vi "GetPaneRefFromLabel.vi"(8 "error in (no error)":errorcluster, 10 "Label":string, 11 "PentaPanesGUI in":refnum<class "PentaPanes.lvclass">) -> (0 "error out":errorcluster, 1 "Index (-1 not found)":i32, 2 "PaneRef":refnum<vi>, 3 "PentaPanesGUI out":refnum<class "PentaPanes.lvclass">)   [LabVIEW 2022 SP3, in "PentaPanesLibrary.lvlib" / "PentaPanes.lvclass"]
doc: "This VI reads the Pane's position string and Label.\n\nPaneRef - A reference to the pane. \nPos String - Outputs a position string (\"Top\", \"Left\", \"Right\", \"Bottom\").\nLabel.Text - Outputs The Label of the pane."
uses:
  PentaPanes.lvclass
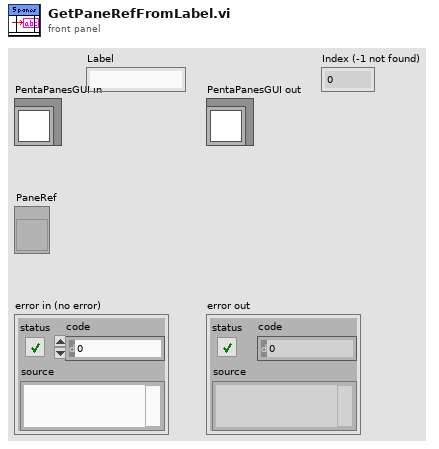
[diagram p1: front panel]
types:
  T1 = typedef "PentaPanesLibrary.lvlib/PentaPanes.lvclass/PanesCluster.ctl" = cluster{"Top Pane":refnum<vi>, "Left Pane":refnum<vi>, "Center Pane":refnum<vi>, "Right Pane":refnum<vi>, "Bottom Pane":refnum<vi>}
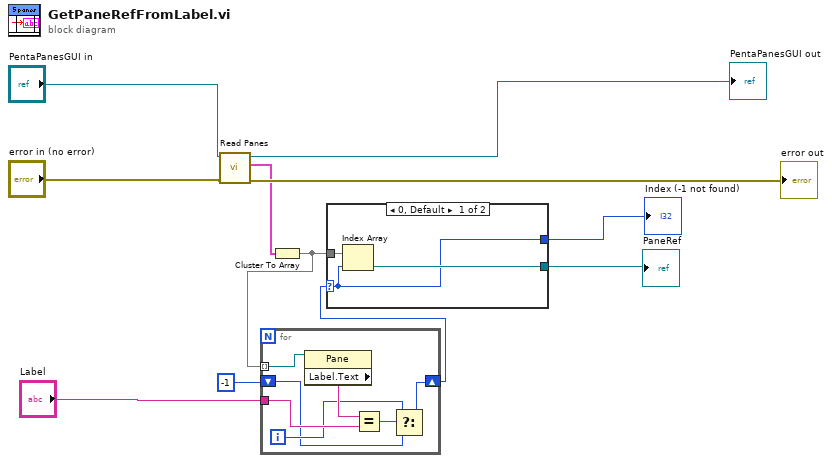
[diagram p0: block diagram]
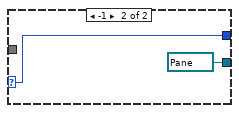
[diagram p2: hidden frame]
diagram:
  n1 = call-dynamic "Read Panes.vi"("error in (no error)"="error in (no error)", "PentaPanesGUI in"="PentaPanesGUI in") -> ("error out"=→"error out":errorcluster, "Panes"=w9:T1, "PentaPanesGUI out"=→"PentaPanesGUI out":refnum<class "PentaPanes.lvclass">)  [unwired: 7 in]
  n2 = Cluster To Array(cluster=w9) -> (array=w6:refnum<vi>[])
  n3 = for {
    tunnel: w6 -> [w18] mode=indexing
    shift-right: [w13] -> w3
    shift-left: -1 -> [w12]
    tunnel: "Label" -> [w16]
    i -> [w14]
    n4 = property class="Pane"(reference=w18) -> ("Label.Text"=w17:string)  [unwired: 1 in, 2 out]
    n5 = Equal?(x=w17, y=w16) -> (x = y?=w15:bool)
    n6 = Select(t=w14, s=w15, f=w12) -> (s? t:f=w13:i32)
  }
  n7 = case shown="0, Default" w3 {
    selector: w3 -> [w19 w22]
    tunnel: w6 -> [w21 _]
    tunnel: [w20 refnum<vi> refnum ("Top Pane")] -> w2
    tunnel: [w19 w22] -> w1
    frame 0, Default {
      n8 = Index Array(array=w21, index=w19) -> (element=w20:refnum<vi>)
    }
    frame -1 {
    }
  }
  "PaneRef" <- w2
  "Index (-1 not found)" <- w1
